vi "Impureza_v0.1.vi"(0 "Image In":T1, 1 "Image Dst":T1, 7 "error in":errorcluster) -> (20 "Image Out":T1, 22 "Reprovado":bool, 27 "error out":errorcluster)   [LabVIEW 2020]
doc: "Creates, edits, and runs vision algorithms using NI Vision Assistant.\n\nWhen you place this Express VI on the block diagram, NI Vision Assistant launches. Create an algorithm using the Vision Assistant processing functions. After you create an algorithm, you can select the controls and indicators that you want to be able to programmatically set in LabVIEW. Double-click the Vision Assistant Express VI to edit the algorithm."
uses:
  <vilib>/vision/Image Controls.llb/IMAQ Image.ctl
  <vilib>/vision/NI_Vision_Development_Module.lvlib
panel:
  out "x > 0? 9":bool
  out "x > 0? 8":bool
  out "x > 0? 7":bool
  out "x > 0? 6":bool
  out "x > 0? 5":bool
  out "x > 0? 4":bool
  out "x > 0? 3":bool
  out "x > 0? 2":bool
  out "x > 0?":bool
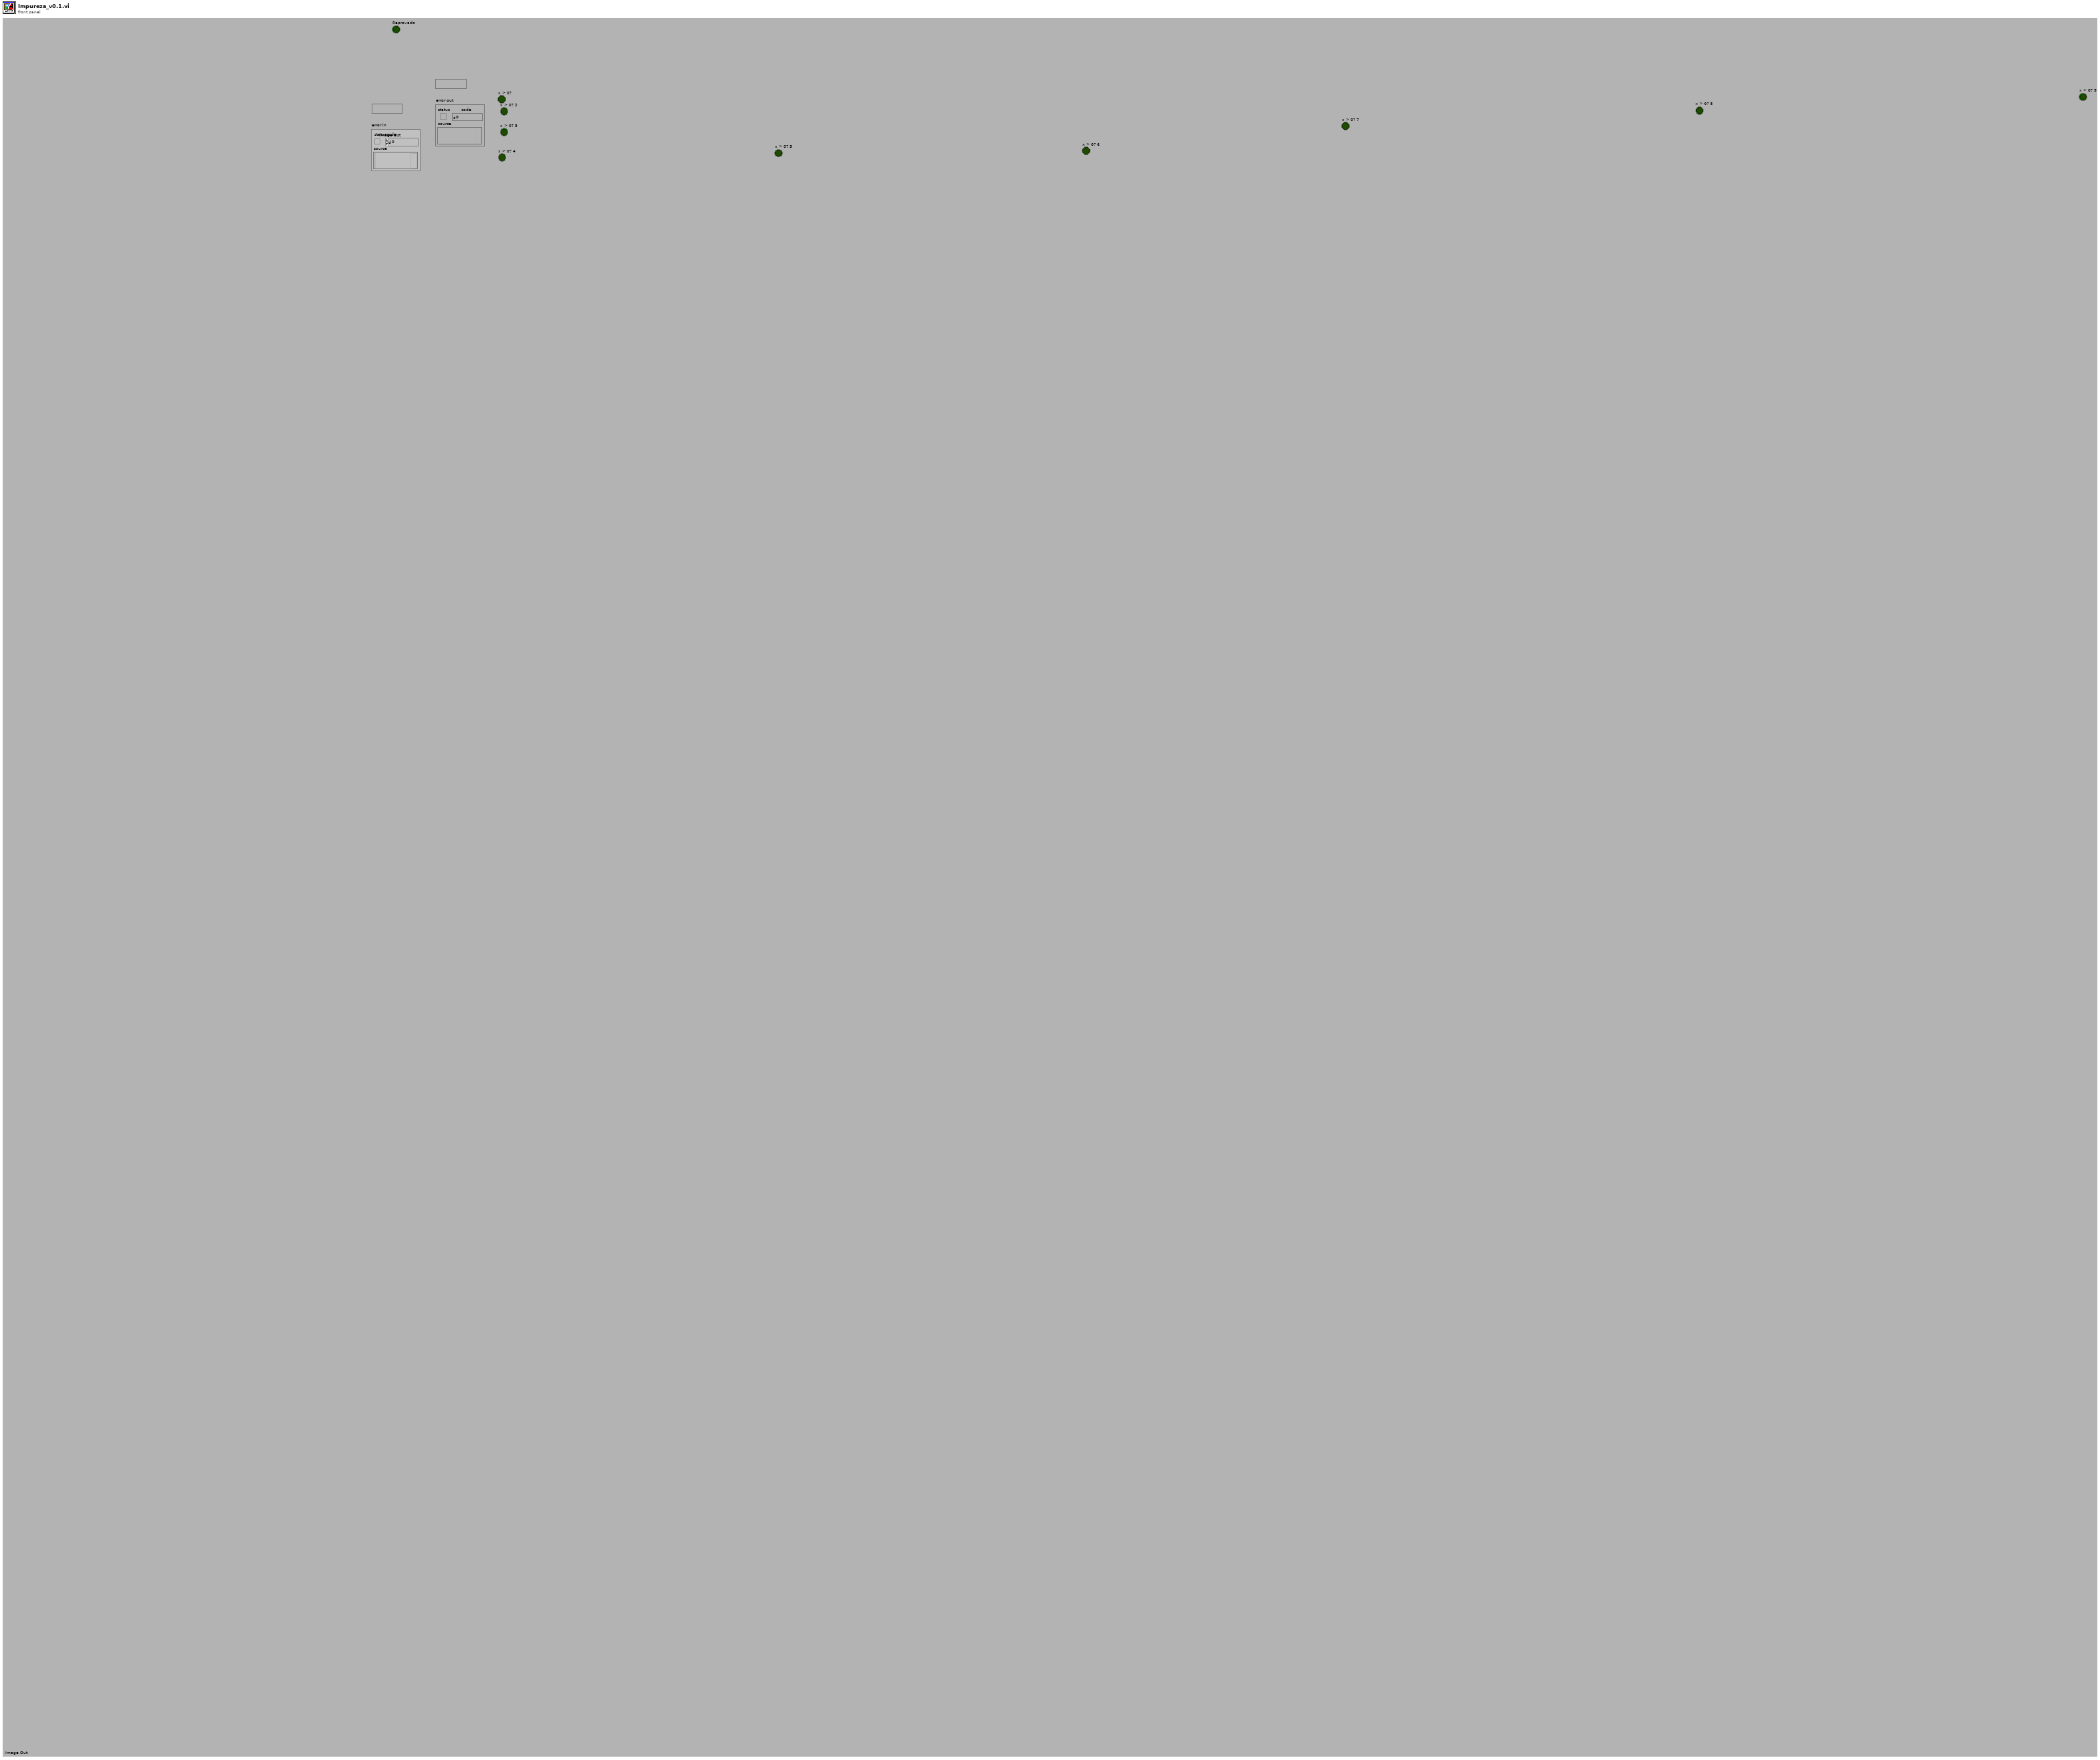
[diagram p1: front panel]
types:
  T1 = typedef "IMAQ Image.ctl" = refnum<image>
  T2 = cluster{"Edge Polarity":u32, "Kernel Size":u32, "Width":u32, "Minimum Edge Strength":sgl, "Interpolation Type":enum32{"Zero Order", "Bilinear", "Quadratic", "Cubic", "Bilinear Fixed"}, "Data Processing Method":enum32{"Average", "Median"}}
  T3 = enum16{"Get First Edge", "Get First + Last Edge", "Get All Edges", "Get Best Edge"}
  T4 = cluster{"Global Rectangle":i32[], "Contours":cluster{"ID":enum32{"External", "Internal"}, "Type":u32, "Coordinates":i32[]}[]}
  T5 = typedef "Image Type" = u32
  T6 = typedef "Edge New.ctl" = cluster{"Location (Pixel)":cluster{"X":sgl, "Y":sgl}, "Location (Real-World)":cluster{"X":sgl, "Y":sgl}, "Distance (Pixel)":dbl, "Distance (Real-World)":dbl, "Strength":dbl, "Noise":dbl, "Rising?":bool}
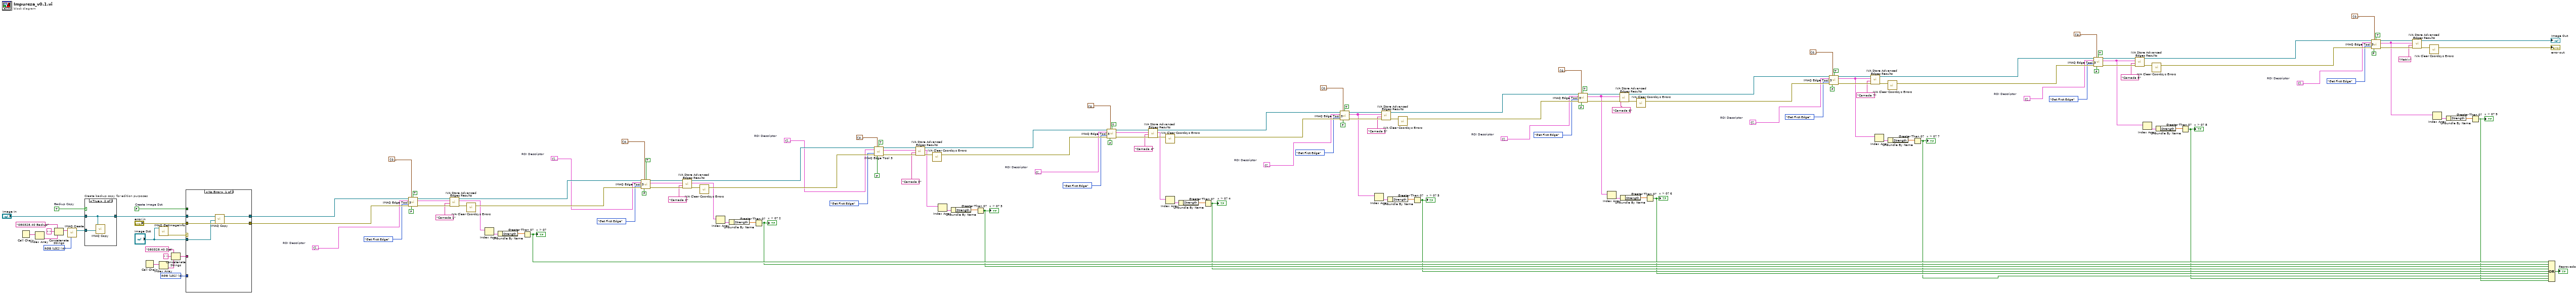
[diagram p0: block diagram]
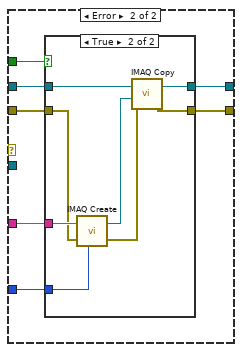
[diagram p2: hidden frame]
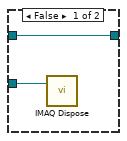
[diagram p4: hidden frame]
diagram:
  w44 = T4 {"Global Rectangle"=[672, 474, 711, 497], "Contours"=[{"ID"=enum."External", "Type"=5, "Coordinates"=[672, 474, 710, 474, 672, 496, 675, 474, 710, 496, 705, 474, 673, 478, 710, 481, 701, 495, 672, 493, 691, 484, 696, 475, 699, 490, 683, 490, 674, 483, 684, 480, 692, 482, 706, 486, 674, 483, 672, 474]}]}  # ROI Descriptor
  w55 = T4 {"Global Rectangle"=[670, 473, 713, 498], "Contours"=[{"ID"=enum."External", "Type"=3, "Coordinates"=[670, 473, 713, 498]}]}  # ROI Descriptor
  w66 = T4 {"Global Rectangle"=[666, 467, 718, 503], "Contours"=[{"ID"=enum."External", "Type"=3, "Coordinates"=[666, 467, 718, 503]}]}  # ROI Descriptor
  w77 = T4 {"Global Rectangle"=[659, 460, 721, 507], "Contours"=[{"ID"=enum."External", "Type"=3, "Coordinates"=[659, 460, 721, 507]}]}  # ROI Descriptor
  w88 = T4 {"Global Rectangle"=[652, 453, 725, 512], "Contours"=[{"ID"=enum."External", "Type"=3, "Coordinates"=[652, 453, 725, 512]}]}  # ROI Descriptor
  w99 = T4 {"Global Rectangle"=[648, 447, 733, 522], "Contours"=[{"ID"=enum."External", "Type"=3, "Coordinates"=[648, 447, 733, 522]}]}  # ROI Descriptor
  w111 = T4 {"Global Rectangle"=[643, 442, 742, 531], "Contours"=[{"ID"=enum."External", "Type"=3, "Coordinates"=[643, 442, 742, 531]}]}  # ROI Descriptor
  w123 = T4 {"Global Rectangle"=[635, 434, 745, 534], "Contours"=[{"ID"=enum."External", "Type"=3, "Coordinates"=[635, 434, 745, 534]}]}  # ROI Descriptor
  w135 = T4 {"Global Rectangle"=[629, 426, 750, 538], "Contours"=[{"ID"=enum."External", "Type"=3, "Coordinates"=[629, 426, 750, 538]}]}  # ROI Descriptor
  w142 = T5 4 items=["Grayscale (U8)", "Grayscale (I16)", "Grayscale (SGL)", "Complex (CSG)", "RGB (U32)", "HSL (U32)", "RGB (U64)", "Grayscale (U16)"] ("Image Dst Type")
  w143 = T5 4 items=["Grayscale (U8)", "Grayscale (I16)", "Grayscale (SGL)", "Complex (CSG)", "RGB (U32)", "HSL (U32)", "RGB (U64)", "Grayscale (U16)"] ("Image Type")
  w162 = TRUE  # Backup Copy
  w155 = FALSE  # Create Image Dst
  n1 = Call Chain() -> (call chain=w149:string[])
  n2 = Index Array(array=w149) -> (element=w148:string)  [unwired: 1 in]
  n3 = Concatenate Strings("080328,40 Backup" ("Backup Image Name"), " ", w148) -> (w145:string)
  n4 = call "IMAQ Create"("Image Name"=w145, "Image Type"=w143) -> ("New Image"=w144:T1)  [unwired: 2 in, 2 out]
  n5 = case "Create backup copy for edition purposes" shown="True" w162 {
    tunnel: [w164 w166] -> w158
    tunnel: "Image In" -> [w164 w166]
    tunnel: w144 -> [w163 w165]
    frame False {
      n6 = call "IMAQ Dispose"("Image"=w163) -> ()  [unwired: 2 in, 4 out]
    }
    frame True {
      n7 = call "IMAQ Copy"("Image Dst"=w165, "Image Src"=w166) -> ()  [unwired: 1 in, 5 out]
    }
  }
  n8 = Call Chain() -> (call chain=w154:string[])
  n9 = call "IMAQ GetImageInfo"("Image"="Image Dst") -> ("error out"=w160:errorcluster)  [unwired: 1 in, 9 out]
  n10 = Index Array(array=w154) -> (element=w152:string)  [unwired: 1 in]
  n11 = Concatenate Strings("080328,40 Dst" ("Image Dst Name"), " ", w152) -> (w150:string)
  n12 = case shown="No Error" w160 {
    tunnel: [w171 w175] -> w141
    tunnel: [w170 w174] -> w156
    tunnel: w158 -> [w169 w176]
    tunnel: "error in" -> [w168 w172]
    tunnel: "Image Dst" -> [w167 _]
    tunnel: w150 -> [_ w178]
    tunnel: w142 -> [_ w177]
    tunnel: w155 -> [_ w173]
    frame No Error {
      n13 = call "IMAQ Copy"("error in (no error)"=w168, "Image Dst"=w167, "Image Src"=w169) -> ("error out"=w170:errorcluster, "Image Dst Out"=w171:T1)  [unwired: 3 out]
    }
    frame Error {
      n14 = case shown="True" w173 {
        tunnel: w178 -> [_ w188]
        tunnel: w177 -> [_ w187]
        tunnel: w176 -> [w180 w185]
        tunnel: [w180 w184] -> w175
        tunnel: [w179 w183] -> w174
        tunnel: w172 -> [w179 w181]
        frame False {
        }
        frame True {
          n15 = call "IMAQ Create"("Image Name"=w188, "Image Type"=w187, "error in (no error)"=w181) -> ("New Image"=w186:T1, "error out"=w182:errorcluster)  [unwired: 1 in, 1 out]
          n16 = call "IMAQ Copy"("error in (no error)"=w182, "Image Dst"=w186, "Image Src"=w185) -> ("error out"=w183:errorcluster, "Image Dst Out"=w184:T1)  [unwired: 3 out]
        }
      }
    }
  }
  n17 = call "IMAQ Edge Tool 3"("Image"=w141, "Edge Options"=T2 {"Edge Polarity"=0, "Kernel Size"=3, "Width"=3, "Minimum Edge Strength"=5.0, "Interpolation Type"=enum."Bilinear Fixed", "Data Processing Method"=enum."Average"}, "Optimized Mode"=TRUE, "ROI Descriptor"=w135, "Process"=T3."Get First Edge", "error in (no error)"=w156, "Reverse Direction"=FALSE) -> ("Image (duplicate)"=w137:T1, "Edge Information"=w38:T6[], "error out"=w138:errorcluster)  [unwired: 6 out]
  n18 = call <vilib>:"IVA Store Advanced Edges Results.vi"("error in (no error)"=w138, "Step Name"="Camada 1", "Edge Information"=w38, "Image in"=w137) -> ("error out"=w132:errorcluster, "Edge Information dup"=w37:T6[], "Image dup"=w130:T1)  [unwired: 5 out]
  n19 = call <vilib>:"IVA Clear Coordsys Errors.vi"("error in (no error)"=w132) -> ("error out"=w131:errorcluster)  [unwired: 10 in]
  n20 = Index Array(array=w37) -> (element=w36:T6)  [unwired: 1 in]
  n21 = Unbundle By Name(w36) -> ("Strength"=w35:dbl)
  n22 = Greater Than 0?(x=w35) -> (x > 0?=w10:bool)
  "x > 0?" <- w10
  n23 = call "IMAQ Edge Tool 3"("Image"=w130, "Edge Options"=T2 {"Edge Polarity"=0, "Kernel Size"=3, "Width"=3, "Minimum Edge Strength"=5.0, "Interpolation Type"=enum."Bilinear Fixed", "Data Processing Method"=enum."Average"}, "Optimized Mode"=TRUE, "ROI Descriptor"=w123, "Process"=T3."Get First Edge", "error in (no error)"=w131, "Reverse Direction"=FALSE) -> ("Image (duplicate)"=w126:T1, "Edge Information"=w125:T6[], "error out"=w127:errorcluster)  [unwired: 6 out]
  n24 = call <vilib>:"IVA Store Advanced Edges Results.vi"("error in (no error)"=w127, "Step Name"="Camada 2", "Edge Information"=w125, "Image in"=w126) -> ("error out"=w120:errorcluster, "Edge Information dup"=w28:T6[], "Image dup"=w118:T1)  [unwired: 5 out]
  n25 = call <vilib>:"IVA Clear Coordsys Errors.vi"("error in (no error)"=w120) -> ("error out"=w119:errorcluster)  [unwired: 10 in]
  n26 = Index Array(array=w28) -> (element=w33:T6)  [unwired: 1 in]
  n27 = Unbundle By Name(w33) -> ("Strength"=w34:dbl)
  n28 = Greater Than 0?(x=w34) -> (x > 0?=w9:bool)
  "x > 0? 2" <- w9
  n29 = call "IMAQ Edge Tool 3"("Image"=w118, "Edge Options"=T2 {"Edge Polarity"=0, "Kernel Size"=3, "Width"=3, "Minimum Edge Strength"=5.0, "Interpolation Type"=enum."Bilinear Fixed", "Data Processing Method"=enum."Average"}, "Optimized Mode"=TRUE, "ROI Descriptor"=w111, "Process"=T3."Get First Edge", "error in (no error)"=w119, "Reverse Direction"=FALSE) -> ("Image (duplicate)"=w114:T1, "Edge Information"=w113:T6[], "error out"=w115:errorcluster)  [unwired: 6 out]
  n30 = call <vilib>:"IVA Store Advanced Edges Results.vi"("error in (no error)"=w115, "Step Name"="Camada 3", "Edge Information"=w113, "Image in"=w114) -> ("error out"=w108:errorcluster, "Edge Information dup"=w27:T6[], "Image dup"=w106:T1)  [unwired: 5 out]
  n31 = call <vilib>:"IVA Clear Coordsys Errors.vi"("error in (no error)"=w108) -> ("error out"=w107:errorcluster)  [unwired: 10 in]
  n32 = Index Array(array=w27) -> (element=w32:T6)  [unwired: 1 in]
  n33 = Unbundle By Name(w32) -> ("Strength"=w31:dbl)
  n34 = Greater Than 0?(x=w31) -> (x > 0?=w8:bool)
  "x > 0? 3" <- w8
  n35 = call "IMAQ Edge Tool 3"("Image"=w106, "Edge Options"=T2 {"Edge Polarity"=0, "Kernel Size"=3, "Width"=3, "Minimum Edge Strength"=5.0, "Interpolation Type"=enum."Bilinear Fixed", "Data Processing Method"=enum."Average"}, "Optimized Mode"=TRUE, "ROI Descriptor"=w99, "Process"=T3."Get First Edge", "error in (no error)"=w107, "Reverse Direction"=FALSE) -> ("Image (duplicate)"=w102:T1, "Edge Information"=w101:T6[], "error out"=w103:errorcluster)  [unwired: 6 out]
  n36 = call <vilib>:"IVA Store Advanced Edges Results.vi"("error in (no error)"=w103, "Step Name"="Camada 4", "Edge Information"=w101, "Image in"=w102) -> ("error out"=w96:errorcluster, "Edge Information dup"=w26:T6[], "Image dup"=w94:T1)  [unwired: 5 out]
  n37 = call <vilib>:"IVA Clear Coordsys Errors.vi"("error in (no error)"=w96) -> ("error out"=w95:errorcluster)  [unwired: 10 in]
  n38 = Index Array(array=w26) -> (element=w29:T6)  [unwired: 1 in]
  n39 = Unbundle By Name(w29) -> ("Strength"=w30:dbl)
  n40 = Greater Than 0?(x=w30) -> (x > 0?=w7:bool)
  "x > 0? 4" <- w7
  n41 = call "IMAQ Edge Tool 3"("Image"=w94, "Edge Options"=T2 {"Edge Polarity"=0, "Kernel Size"=3, "Width"=3, "Minimum Edge Strength"=5.0, "Interpolation Type"=enum."Bilinear Fixed", "Data Processing Method"=enum."Average"}, "Optimized Mode"=TRUE, "ROI Descriptor"=w88, "Process"=T3."Get First Edge", "error in (no error)"=w95, "Reverse Direction"=FALSE) -> ("Image (duplicate)"=w90:T1, "Edge Information"=w15:T6[], "error out"=w91:errorcluster)  [unwired: 6 out]
  n42 = Index Array(array=w15) -> (element=w25:T6)  [unwired: 1 in]
  n43 = call <vilib>:"IVA Store Advanced Edges Results.vi"("error in (no error)"=w91, "Step Name"="Camada 5", "Edge Information"=w15, "Image in"=w90) -> ("error out"=w85:errorcluster, "Image dup"=w83:T1)  [unwired: 6 out]
  n44 = Unbundle By Name(w25) -> ("Strength"=w24:dbl)
  n45 = call <vilib>:"IVA Clear Coordsys Errors.vi"("error in (no error)"=w85) -> ("error out"=w84:errorcluster)  [unwired: 10 in]
  n46 = Greater Than 0?(x=w24) -> (x > 0?=w6:bool)
  "x > 0? 5" <- w6
  n47 = call "IMAQ Edge Tool 3"("Image"=w83, "Edge Options"=T2 {"Edge Polarity"=0, "Kernel Size"=3, "Width"=3, "Minimum Edge Strength"=5.0, "Interpolation Type"=enum."Bilinear Fixed", "Data Processing Method"=enum."Average"}, "Optimized Mode"=TRUE, "ROI Descriptor"=w77, "Process"=T3."Get First Edge", "error in (no error)"=w84, "Reverse Direction"=FALSE) -> ("Image (duplicate)"=w79:T1, "Edge Information"=w14:T6[], "error out"=w80:errorcluster)  [unwired: 6 out]
  n48 = Index Array(array=w14) -> (element=w22:T6)  [unwired: 1 in]
  n49 = call <vilib>:"IVA Store Advanced Edges Results.vi"("error in (no error)"=w80, "Step Name"="Camada 6", "Edge Information"=w14, "Image in"=w79) -> ("error out"=w74:errorcluster, "Image dup"=w72:T1)  [unwired: 6 out]
  n50 = Unbundle By Name(w22) -> ("Strength"=w23:dbl)
  n51 = call <vilib>:"IVA Clear Coordsys Errors.vi"("error in (no error)"=w74) -> ("error out"=w73:errorcluster)  [unwired: 10 in]
  n52 = Greater Than 0?(x=w23) -> (x > 0?=w5:bool)
  "x > 0? 6" <- w5
  n53 = call "IMAQ Edge Tool 3"("Image"=w72, "Edge Options"=T2 {"Edge Polarity"=0, "Kernel Size"=3, "Width"=3, "Minimum Edge Strength"=5.0, "Interpolation Type"=enum."Bilinear Fixed", "Data Processing Method"=enum."Average"}, "Optimized Mode"=TRUE, "ROI Descriptor"=w66, "Process"=T3."Get First Edge", "error in (no error)"=w73, "Reverse Direction"=FALSE) -> ("Image (duplicate)"=w68:T1, "Edge Information"=w13:T6[], "error out"=w69:errorcluster)  [unwired: 6 out]
  n54 = call <vilib>:"IVA Store Advanced Edges Results.vi"("error in (no error)"=w69, "Step Name"="Camada 7", "Edge Information"=w13, "Image in"=w68) -> ("error out"=w63:errorcluster, "Image dup"=w61:T1)  [unwired: 6 out]
  n55 = Index Array(array=w13) -> (element=w21:T6)  [unwired: 1 in]
  n56 = call <vilib>:"IVA Clear Coordsys Errors.vi"("error in (no error)"=w63) -> ("error out"=w62:errorcluster)  [unwired: 10 in]
  n57 = Unbundle By Name(w21) -> ("Strength"=w20:dbl)
  n58 = Greater Than 0?(x=w20) -> (x > 0?=w4:bool)
  "x > 0? 7" <- w4
  n59 = call "IMAQ Edge Tool 3"("Image"=w61, "Edge Options"=T2 {"Edge Polarity"=0, "Kernel Size"=3, "Width"=3, "Minimum Edge Strength"=5.0, "Interpolation Type"=enum."Bilinear Fixed", "Data Processing Method"=enum."Average"}, "Optimized Mode"=TRUE, "ROI Descriptor"=w55, "Process"=T3."Get First Edge", "error in (no error)"=w62, "Reverse Direction"=FALSE) -> ("Image (duplicate)"=w57:T1, "Edge Information"=w12:T6[], "error out"=w58:errorcluster)  [unwired: 6 out]
  n60 = call <vilib>:"IVA Store Advanced Edges Results.vi"("error in (no error)"=w58, "Step Name"="Camada 8", "Edge Information"=w12, "Image in"=w57) -> ("error out"=w52:errorcluster, "Image dup"=w50:T1)  [unwired: 6 out]
  n61 = Index Array(array=w12) -> (element=w18:T6)  [unwired: 1 in]
  n62 = call <vilib>:"IVA Clear Coordsys Errors.vi"("error in (no error)"=w52) -> ("error out"=w51:errorcluster)  [unwired: 10 in]
  n63 = Unbundle By Name(w18) -> ("Strength"=w19:dbl)
  n64 = Greater Than 0?(x=w19) -> (x > 0?=w3:bool)
  "x > 0? 8" <- w3
  n65 = call "IMAQ Edge Tool 3"("Image"=w50, "Edge Options"=T2 {"Edge Polarity"=0, "Kernel Size"=3, "Width"=3, "Minimum Edge Strength"=5.0, "Interpolation Type"=enum."Bilinear Fixed", "Data Processing Method"=enum."Average"}, "Optimized Mode"=TRUE, "ROI Descriptor"=w44, "Process"=T3."Get First Edge", "error in (no error)"=w51, "Reverse Direction"=FALSE) -> ("Image (duplicate)"=w46:T1, "Edge Information"=w11:T6[], "error out"=w47:errorcluster)  [unwired: 6 out]
  n66 = call <vilib>:"IVA Store Advanced Edges Results.vi"("error in (no error)"=w47, "Step Name"="Matrix", "Edge Information"=w11, "Image in"=w46) -> ("error out"=w41:errorcluster, "Image dup"=→"Image Out":T1)  [unwired: 6 out]
  n67 = call <vilib>:"IVA Clear Coordsys Errors.vi"("error in (no error)"=w41) -> ("error out"=→"error out":errorcluster)  [unwired: 10 in]
  n68 = Index Array(array=w11) -> (element=w17:T6)  [unwired: 1 in]
  n69 = Unbundle By Name(w17) -> ("Strength"=w16:dbl)
  n70 = Greater Than 0?(x=w16) -> (x > 0?=w2:bool)
  "x > 0? 9" <- w2
  n71 = Compound Arithmetic op=OR(w10, w9, w8, w7, w6, w5, w4, w3, w2) -> (→"Reprovado":bool)
